vi "EditorSub createPyScript.vi"(0 "newScriptCode":string) -> (1 "scriptStartIdx":i32, 2 "pyCode":string)   [LabVIEW 2018]
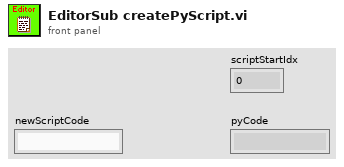
[diagram p1: front panel]
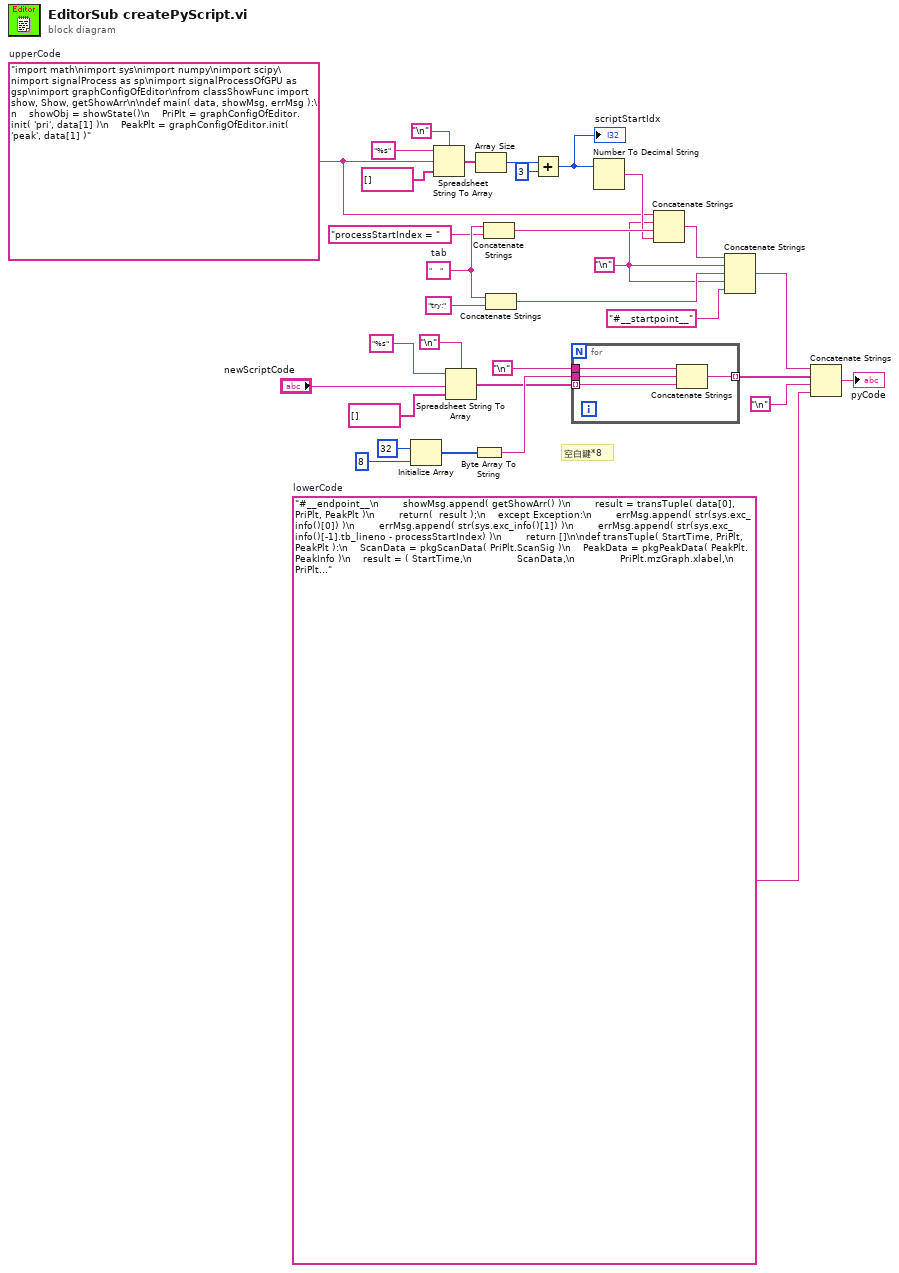
[diagram p0: block diagram]
diagram:
  w13 = "    "  # tab
  w5 = "\n"
  w4 = "#__endpoint__\n        showMsg.append( getShowArr() )\n        result = transTuple( data[0], PriPlt, PeakPlt )\n        return(  result );\n    except Exception:\n        errMsg.append( str(sys.exc_info()[0]) )\n        errMsg.append( str(sys.exc_info()[1]) )\n        errMsg.append( str(sys.exc_info()[-1].tb_lineno - processStartIndex) )\n        return []\n\ndef transTuple( StartTime, PriPlt, PeakPlt ):\n    ScanData = pkgScanData( PriPlt.ScanSig )\n    PeakData = pkgPeakData( PeakPlt.PeakInfo )\n    result = ( StartTime,\n               ScanData,\n               PriPlt.mzGraph.xlabel,\n               PriPlt.mzGraph.ylabel,\n               PeakData )\n    return result\n\n### package scan data\ndef pkgScanData( data ):\n    scanData=[]\n    for sig in data:\n        if type( sig.xdata ) != list:\n            sig.xdata = sig.xdata.tolist()\n        if type( sig.ydata ) != list:\n            sig.ydata = sig.ydata.tolist()\n        if type( sig.beta ) != list:\n            sig.beta = sig.beta.tolist()\n        scanTuple = ( sig.dt, sig.xdata, sig.ydata, sig.beta ) \n        scanData.append( scanTuple )\n    return scanData\n\n### package peak information data\ndef pkgPeakData( data ):\n    peakData=[]\n    for sig in data:\n        if type( sig.xLdata ) != list:\n            sig.xLdata = sig.xLdata.tolist()\n        if type( sig.xCdata ) != list:\n            sig.xCdata = sig.xCdata.tolist()\n        if type( sig.xRdata ) != list:\n            sig.xRdata = sig.xRdata.tolist()\n        if type( sig.baseline ) != list:\n            sig.baseline = sig.baseline.tolist()\n        if type( sig.halfHeight ) != list:\n            sig.halfHeight = sig.halfHeight.tolist()\n        peakTuple = ( sig.xLdata, sig.xCdata, sig.xRdata, sig.baseline, sig.halfHeight )\n        peakData.append( peakTuple )\n    return peakData"  # lowerCode
  w2 = "import math\nimport sys\nimport numpy\nimport scipy\nimport signalProcess as sp\nimport signalProcessOfGPU as gsp\nimport graphConfigOfEditor\nfrom classShowFunc import show, Show, getShowArr\n\ndef main( data, showMsg, errMsg ):\n    showObj = showState()\n    PriPlt = graphConfigOfEditor.init( 'pri', data[1] )\n    PeakPlt = graphConfigOfEditor.init( 'peak', data[1] )"  # upperCode
  # "空白鍵*8"
  n1 = Initialize Array(u8 32, 8 ("dimension size")) -> (w29:u8[])
  n2 = Spreadsheet String To Array(delimiter (Tab)="\n", format string="%s", spreadsheet string=w2, array type (2D Dbl)=string[] []) -> (array=w15:string[])
  n3 = Spreadsheet String To Array(delimiter (Tab)="\n", format string="%s", spreadsheet string="newScriptCode", array type (2D Dbl)=string[] []) -> (array=w24:string[])
  n4 = Byte Array To String(unsigned byte array=w29) -> (string=w28:string)
  n5 = Array Size(array=w15) -> (size(s)=w20:i32)
  n6 = Concatenate Strings(w13, "processStartIndex = " ("string")) -> (w18:string)
  n7 = Concatenate Strings(w13, "try:" ("string")) -> (w19:string)
  n8 = Add(x=w20, y=3) -> (x+y=w21:i32)
  "scriptStartIdx" <- w21
  n9 = for {
    tunnel: w24 -> [w33] mode=indexing
    tunnel: w28 -> [w36]
    tunnel: [w35] -> w23 mode=indexing
    tunnel: "\n" ("delimiter (Tab)") -> [w34]
    n10 = Concatenate Strings(w34, w36, w33) -> (w35:string)
  }
  n11 = Number To Decimal String(number=w21) -> (decimal integer string=w16:string)  [unwired: 1 in]
  n12 = Concatenate Strings(w2, w5, w18, w16) -> (w17:string)
  n13 = Concatenate Strings(w17, w5, w19, w5, "#__startpoint__" ("string")) -> (w7:string)
  n14 = Concatenate Strings(w7, w23, "\n" ("delimiter (Tab)"), w4) -> (→"pyCode":string)
